vi "Configure Constant Voltage.vi"(8 "error in (no error)":errorcluster, 10 "CV Voltage (0.1)":dbl=0.1 min=0.1 max=500.0 step=1.0 format="%#.4g", 11 "VISA resource name":refnum<visa-resource-name>) -> (0 "error out":errorcluster, 3 "VISA resource name out":refnum<visa-resource-name>)   [LabVIEW 2024, in "BK Precision 8500B Series.lvlib"]
doc: "Configures the voltage and current max/min limit for constant voltage (CV) operation."
uses:
  BK Precision 8500B Series.lvlib
panel:
  # "V"
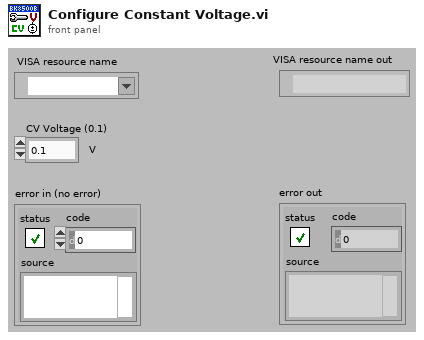
[diagram p1: front panel]
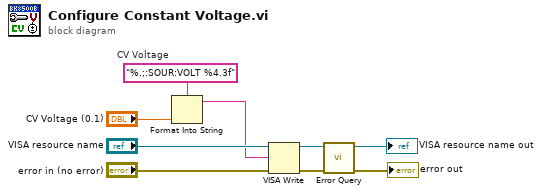
[diagram p0: block diagram]
diagram:
  w7 = "%.;:SOUR:VOLT %4.3f"  # CV Voltage
  n1 = Format Into String(format string=w7, "CV Voltage (0.1)") -> (resulting string=w1:string)  [unwired: 2 in, 1 out]
  n2 = VISA Write(VISA resource name="VISA resource name", write buffer=w1, error in (no error)="error in (no error)") -> (VISA resource name out=w5:refnum<visa-resource-name>, error out=w6:errorcluster)  [unwired: 1 out]
  n3 = call "Error Query.vi"("error in (no error)"=w6, "VISA resource name"=w5) -> ("error out"=→"error out":errorcluster, "VISA resource name out"=→"VISA resource name out":refnum<visa-resource-name>)  [unwired: 6 in, 2 out]
